vi "GetNameVersion.vi"(8 "error in (no error)":errorcluster, 11 "XML String":string="<?xml version=\"1.0\" encoding=\"utf-8\"?>\n<CustomDevice xmlns:xsi=\"http://www.w3.org/2001/XMLSchema-instance\" xsi:noNamespaceSchemaLocation=\"Custom Device.xsd\">\n<XSDVersion Major=\"2010\" Minor=\"0\" Fix=\"0\" Build=\"0\" />\n  <AddMenu>\n    <eng>NI-XNET Monitor</eng>\n    <loc>NI-XNET Monitor</loc>\n  </AddMenu>\n  <Version>2.0.0</Version>\n  <Type>Inline HW Interface</Type>\n  <MaxOccurrence>1</MaxOccurrence>\n  <MainPageGUID>2fba45b0-1589-4179-a966-5fc49498794e</MainPageGUID>\n  <InitializationVI>\n    <Type>Action</Type>\n    <Item2Launch>\n      <Type>To Common Doc Dir</Type>\n\t\t<Path>Custom Devices\\NI-XNET Monitor\\Windows\\NI-XNET Monitor Configuration.llb\\Initialization VI.vi</Path>\n    </Item2Launch>\n  </InitializationVI>\n  <CustomDeviceVI>\n\t\t<SourceDistribution>\n\t\t\t<Source>\n\t\t\t\t<SupportedTarget>Windows</SupportedTarget>\n\t\t\t\t<Source>\n\t\t\t\t\t<Type>To Common Doc Dir</Type>\n\t\t\t\t\t<Path>Custom Devices\\NI-XNET Monitor\\Windows\\NI-XNET Monitor Engine Windows.llb\\RT Driver VI.vi</Path>\n\t\t\t\t</Source>\n\t\t\t\t<RealTimeSystemDestination>c:\\ni-rt\\VeriStand\\Custom Devices\\NI-XNET Monitor\\NI-XNET Monitor Engine Windows.llb\\RT Driver VI.vi</RealTimeSystemDestination>\n\t\t\t</Source>\n\t\t\t<Source>\n\t\t\t\t<SupportedTarget>Pharlap</SupportedTarget>\n\t\t\t\t<Source>\n\t\t\t\t\t<Type>To Common Doc Dir</Type>\n\t\t\t\t\t<Path>Custom Devices\\NI-XNET Monitor\\PharLap\\NI-XNET Monitor Engine Pharlap.llb\\RT Driver VI.vi</Path>\n\t\t\t\t</Source>\n\t\t\t\t<RealTimeSystemDestination>c:\\ni-rt\\VeriStand\\Custom Devices\\NI-XNET Monitor\\NI-XNET Monitor Engine Pharlap.llb\\RT Driver VI.vi</RealTimeSystemDestination>\n\t\t\t</Source>\n\t\t\t<Source>\n\t\t\t\t<SupportedTarget>VxWorks</SupportedTarget>\n\t\t\t\t<Source>\n\t\t\t\t\t<Type>To Common Doc Dir</Type>\n\t\t\t\t\t<Path>Custom Devices\\NI-XNET Monitor\\VxWorks\\NI-XNET Monitor Engine VxWorks.llb\\RT Driver VI.vi</Path>\n\t\t\t\t</Source>\n\t\t\t\t<RealTimeSystemDestination>c:\\ni-rt\\VeriStand\\Custom Devices\\NI-XNET Monitor\\NI-XNET Monitor Engine VxWorks.llb\\RT Driver VI.vi</RealTimeSystemDestination>\n\t\t\t</Source>\t\n\t\t\t<Source>\n\t\t\t\t<SupportedTarget>Linux_32_ARM</SupportedTarget>\n\t\t\t\t<Source>\n\t\t\t\t\t<Type>To Common Doc Dir</Type>\n\t\t\t\t\t<Path>Custom Devices\\NI-XNET Monitor\\Linux_32_ARM\\NI-XNET Monitor Engine LinuxARM.llb\\RT Driver VI.vi</Path>\n\t\t\t\t</Source>\n\t\t\t\t<RealTimeSystemDestination>c:\\ni-rt\\VeriStand\\Custom Devices\\NI-XNET Monitor\\NI-XNET Monitor Engine LinuxARM.llb\\RT Driver VI.vi</RealTimeSystemDestination>\n\t\t\t</Source>\n\t\t\t<Source>\n\t\t\t\t<SupportedTarget>Linux_x64</SupportedTarget>\n\t\t\t\t<Source>\n\t\t\t\t\t<Type>To Common Doc Dir</Type>\n\t\t\t\t\t<Path>Custom Devices\\NI-XNET Monitor\\Linux_x64\\NI-XNET Monitor Engine Linux64.llb\\RT Driver VI.vi</Path>\n\t\t\t\t</Source>\n\t\t\t\t<RealTimeSystemDestination>c:\\ni-rt\\VeriStand\\Custom Devices\\NI-XNET Monitor\\NI-XNET Monitor Engine Linux64.llb\\RT Driver VI.vi</RealTimeSystemDestination>\n\t\t\t</Source>\n\t\t</SourceDistribution>\n\t</CustomDeviceVI>\n  <Dependencies />\n  <Pages>\n    <Page>\n      <Name>\n        <eng>NI-XNET Monitor</eng>\n        <loc>NI-XNET Monitor</loc>\n      </Name>\n\t  <DisallowRenaming>true</DisallowRenaming>\n      <GUID>2fba45b0-1589-4179-a966-5fc49498794e</GUID>\n      <Glyph>\n\t\t\t<Type>To Common Doc Dir</Type>\n\t\t\t<Path>Custom Devices\\NI-XNET Monitor\\Glyphs\\xnet_monitor.png</Path>\n\t\t</Glyph>\n      <Item2Launch>\n        <Type>To Common Doc Dir</Type>\n\t\t<Path>Custom Devices\\NI-XNET Monitor\\Windows\\NI-XNET Monitor Configuration.llb\\Main Page.vi</Path>\n      </Item2Launch>\n\t  <ButtonList>\n\t\t\t<Button>\n\t\t\t\t<ID>Refresh-Button</ID>\n\t\t\t\t<Glyph>\n\t\t\t\t\t<Type>To Application Data Dir</Type>\n\t\t\t\t\t<Path>System Explorer\\Glyphs\\reload.png</Path>\n\t\t\t\t</Glyph>\n\t\t\t\t<Type>Notification</Type>\n\t\t\t\t<ReferencedGUID>2fba45b0-1589-4179-a966-5fc49498794e</ReferencedGUID>\n\t\t\t\t<ButtonText>\n\t\t\t\t\t<eng>Refresh</eng>\n\t\t\t\t\t<loc>Refresh</loc>\n\t\t\t\t</ButtonText>\n\t\t\t\t<Caption>\n\t\t\t\t\t<eng>Refresh</eng>\n\t\t\t\t\t<loc>Refresh</loc>\n\t\t\t\t</Caption>\n\t\t\t\t<TipStrip>\n\t\t\t\t\t<eng>Refresh NI-XNET channel list</eng>\n\t\t\t\t\t<loc>Refresh NI-XNET channel list</loc>\n\t\t\t\t</TipStrip>\n\t\t\t\t<Documentation>\n\t\t\t\t\t<eng>Refresh NI-XNET channel list</eng>\n\t\t\t\t\t<loc>Refresh NI-XNET channel list</loc>\n\t\t\t\t</Documentation>\n\t\t\t</Button>\n\t  </ButtonList>\n\t  <ActionVIOnDelete>\n \t\t <Type>To Common Doc Dir</Type>\n\t\t <Path>Custom Devices\\NI-XNET Monitor\\Windows\\NI-XNET Monitor Configuration.llb\\ActionVIOnDelete.vi</Path>\n\t  </ActionVIOnDelete>\n      <ActionVIOnLoad>\n        <Type>To Common Doc Dir</Type>\n        <Path>Custom Devices\\NI-XNET Monitor\\Windows\\NI-XNET Monitor Configuration.llb\\ActionVIOnLoad.vi</Path>\n      </ActionVIOnLoad>\n      <ActionVIOnSave>\n        <Type>To Common Doc Dir</Type>\n        <Path>Custom Devices\\NI-XNET Monitor\\Windows\\NI-XNET Monitor Configuration.llb\\ActionVIOnSave.vi</Path>\n      </ActionVIOnSave>\n\t  <ActionVIOnCompile>\n        <Type>To Common Doc Dir</Type>\n        <Path>Custom Devices\\NI-XNET Monitor\\Windows\\NI-XNET Monitor Configuration.llb\\ActionVIOnCompile.vi</Path>\n      </ActionVIOnCompile>\n    </Page>\n    \n<Page>\n      <Name>\n        <eng>Port</eng>\n        <loc>Port</loc>\n      </Name>\n\t  <DisallowRenaming>true</DisallowRenaming>\n\t  <ExcludeFromAlphabeticalOrder>true</ExcludeFromAlphabeticalOrder>\n      <GUID>6e4b4e9f-3d48-4140-aa73-eb1a9ddd4810</GUID>\n      <Glyph>\n\t\t\t<Type>To Application Data Dir</Type>\n\t\t\t<Path>System Explorer\\Glyphs\\NI-XNET Port.png</Path>\n\t\t</Glyph>\n      <Item2Launch>\n        <Type>To Common Doc Dir</Type>\n\t\t<Path>Custom Devices\\NI-XNET Monitor\\Windows\\NI-XNET Monitor Configuration.llb\\Port.vi</Path>\n      </Item2Launch>\n\t  <ButtonList>\n\t\t\t<Button>\n\t\t\t\t<ID>Refresh-Button</ID>\n\t\t\t\t<Glyph>\n\t\t\t\t\t<Type>To Application Data Dir</Type>\n\t\t\t\t\t<Path>System Explorer\\Glyphs\\reload.png</Path>\n\t\t\t\t</Glyph>\n\t\t\t\t<Type>Notification</Type>\n\t\t\t\t<ReferencedGUID>6e4b4e9f-3d48-4140-aa73-eb1a9ddd4810</ReferencedGUID>\n\t\t\t\t<ButtonText>\n\t\t\t\t\t<eng>Refresh</eng>\n\t\t\t\t\t<loc>Refresh</loc>\n\t\t\t\t</ButtonText>\n\t\t\t\t<Caption>\n\t\t\t\t\t<eng>Refresh</eng>\n\t\t\t\t\t<loc>Refresh</loc>\n\t\t\t\t</Caption>\n\t\t\t\t<TipStrip>\n\t\t\t\t\t<eng>Refresh NI-XNET channel list</eng>\n\t\t\t\t\t<loc>Refresh NI-XNET channel list</loc>\n\t\t\t\t</TipStrip>\n\t\t\t\t<Documentation>\n\t\t\t\t\t<eng>Refresh NI-XNET channel list</eng>\n\t\t\t\t\t<loc>Refresh NI-XNET channel list</loc>\n\t\t\t\t</Documentation>\n\t\t\t</Button>\n\t  </ButtonList>\n    </Page>\n<Page>\n      <Name>\n        <eng>Port</eng>\n        <loc>Port</loc>\n      </Name>\n\t  <DisallowRenaming>true</DisallowRenaming>\n\t  <ExcludeFromAlphabeticalOrder>true</ExcludeFromAlphabeticalOrder>\n      <GUID>6e4b4e9f-3d48-4140-aa73-eb1a9ddd4810-DISABLED</GUID>\n      <Glyph>\n\t\t\t<Type>To Application Data Dir</Type>\n\t\t\t<Path>System Explorer\\Glyphs\\NI-XNET Port Disabled.png</Path>\n\t\t</Glyph>\n      <Item2Launch>\n        <Type>To Common Doc Dir</Type>\n\t\t<Path>Custom Devices\\NI-XNET Monitor\\Windows\\NI-XNET Monitor Configuration.llb\\Port.vi</Path>\n      </Item2Launch>\n\t  <ButtonList>\n\t\t\t<Button>\n\t\t\t\t<ID>Refresh-Button</ID>\n\t\t\t\t<Glyph>\n\t\t\t\t\t<Type>To Application Data Dir</Type>\n\t\t\t\t\t<Path>System Explorer\\Glyphs\\reload.png</Path>\n\t\t\t\t</Glyph>\n\t\t\t\t<Type>Notification</Type>\n\t\t\t\t<ReferencedGUID>6e4b4e9f-3d48-4140-aa73-eb1a9ddd4810-DISABLED</ReferencedGUID>\n\t\t\t\t<ButtonText>\n\t\t\t\t\t<eng>Refresh</eng>\n\t\t\t\t\t<loc>Refresh</loc>\n\t\t\t\t</ButtonText>\n\t\t\t\t<Caption>\n\t\t\t\t\t<eng>Refresh</eng>\n\t\t\t\t\t<loc>Refresh</loc>\n\t\t\t\t</Caption>\n\t\t\t\t<TipStrip>\n\t\t\t\t\t<eng>Refresh NI-XNET channel list</eng>\n\t\t\t\t\t<loc>Refresh NI-XNET channel list</loc>\n\t\t\t\t</TipStrip>\n\t\t\t\t<Documentation>\n\t\t\t\t\t<eng>Refresh NI-XNET channel list</eng>\n\t\t\t\t\t<loc>Refresh NI-XNET channel list</loc>\n\t\t\t\t</Documentation>\n\t\t\t</Button>\n\t  </ButtonList>\n    </Page>\n<Page>\n      <Name>\n        <eng>CAN</eng>\n        <loc>CAN</loc>\n      </Name>\n\t  <DisallowRenaming>true</DisallowRenaming>\n\t  <ExcludeFromAlphabeticalOrder>true</ExcludeFromAlphabeticalOrder>\n      <GUID>d0ed4327-8d71-4af7-8daf-159d159a2198</GUID>\n      <Glyph>\n\t\t\t<Type>To Application Data Dir</Type>\n\t\t\t<Path>System Explorer\\Glyphs\\NI-XNET CAN.png</Path>\n\t\t</Glyph>\n      <Item2Launch>\n        <Type>To Common Doc Dir</Type>\n\t\t<Path>Custom Devices\\NI-XNET Monitor\\Windows\\NI-XNET Monitor Configuration.llb\\Interface.vi</Path>\n      </Item2Launch>\n\t  <ButtonList>\n\t\t\t<Button>\n\t\t\t\t<ID>Refresh-Button</ID>\n\t\t\t\t<Glyph>\n\t\t\t\t\t<Type>To Application Data Dir</Type>\n\t\t\t\t\t<Path>System Explorer\\Glyphs\\reload.png</Path>\n\t\t\t\t</Glyph>\n\t\t\t\t<Type>Notification</Type>\n\t\t\t\t<ReferencedGUID>d0ed4327-8d71-4af7-8daf-159d159a2198</ReferencedGUID>\n\t\t\t\t<ButtonText>\n\t\t\t\t\t<eng>Refresh</eng>\n\t\t\t\t\t<loc>Refresh</loc>\n\t\t\t\t</ButtonText>\n\t\t\t\t<Caption>\n\t\t\t\t\t<eng>Refresh</eng>\n\t\t\t\t\t<loc>Refresh</loc>\n\t\t\t\t</Caption>\n\t\t\t\t<TipStrip>\n\t\t\t\t\t<eng>Refresh NI-XNET channel list</eng>\n\t\t\t\t\t<loc>Refresh NI-XNET channel list</loc>\n\t\t\t\t</TipStrip>\n\t\t\t\t<Documentation>\n\t\t\t\t\t<eng>Refresh NI-XNET channel list</eng>\n\t\t\t\t\t<loc>Refresh NI-XNET channel list</loc>\n\t\t\t\t</Documentation>\n\t\t\t</Button>\n\t  </ButtonList>\n    </Page>\n<Page>\n      <Name>\n        <eng>FlexRay</eng>\n        <loc>FlexRay</loc>\n      </Name>\n\t  <DisallowRenaming>true</DisallowRenaming>\n\t  <ExcludeFromAlphabeticalOrder>true</ExcludeFromAlphabeticalOrder>\n      <GUID>b3b15e68-7151-4c2d-a280-06a82878b967</GUID>\n      <Glyph>\n\t\t\t<Type>To Application Data Dir</Type>\n\t\t\t<Path>System Explorer\\Glyphs\\NI-XNET FlexRay.png</Path>\n\t\t</Glyph>\n      <Item2Launch>\n        <Type>To Common Doc Dir</Type>\n\t\t<Path>Custom Devices\\NI-XNET Monitor\\Windows\\NI-XNET Monitor Configuration.llb\\Interface.vi</Path>\n      </Item2Launch>\n\t  <ButtonList>\n\t\t\t<Button>\n\t\t\t\t<ID>Refresh-Button</ID>\n\t\t\t\t<Glyph>\n\t\t\t\t\t<Type>To Application Data Dir</Type>\n\t\t\t\t\t<Path>System Explorer\\Glyphs\\reload.png</Path>\n\t\t\t\t</Glyph>\n\t\t\t\t<Type>Notification</Type>\n\t\t\t\t<ReferencedGUID>b3b15e68-7151-4c2d-a280-06a82878b967</ReferencedGUID>\n\t\t\t\t<ButtonText>\n\t\t\t\t\t<eng>Refresh</eng>\n\t\t\t\t\t<loc>Refresh</loc>\n\t\t\t\t</ButtonText>\n\t\t\t\t<Caption>\n\t\t\t\t\t<eng>Refresh</eng>\n\t\t\t\t\t<loc>Refresh</loc>\n\t\t\t\t</Caption>\n\t\t\t\t<TipStrip>\n\t\t\t\t\t<eng>Refresh NI-XNET channel list</eng>\n\t\t\t\t\t<loc>Refresh NI-XNET channel list</loc>\n\t\t\t\t</TipStrip>\n\t\t\t\t<Documentation>\n\t\t\t\t\t<eng>Refresh NI-XNET channel list</eng>\n\t\t\t\t\t<loc>Refresh NI-XNET channel list</loc>\n\t\t\t\t</Documentation>\n\t\t\t</Button>\n\t  </ButtonList>\n    </Page>\n<Page>\n      <Name>\n        <eng>LIN</eng>\n        <loc>LIN</loc>\n      </Name>\n\t  <DisallowRenaming>true</DisallowRenaming>\n\t  <ExcludeFromAlphabeticalOrder>true</ExcludeFromAlphabeticalOrder>\n      <GUID>c19a2e81-5516-4045-93a5-b1bca7ac20ae</GUID>\n      <Glyph>\n\t\t\t<Type>To Application Data Dir</Type>\n\t\t\t<Path>System Explorer\\Glyphs\\NI-XNET LIN.png</Path>\n\t\t</Glyph>\n      <Item2Launch>\n        <Type>To Common Doc Dir</Type>\n\t\t<Path>Custom Devices\\NI-XNET Monitor\\Windows\\NI-XNET Monitor Configuration.llb\\Interface.vi</Path>\n      </Item2Launch>\n\t  <ButtonList>\n\t\t\t<Button>\n\t\t\t\t<ID>Refresh-Button</ID>\n\t\t\t\t<Glyph>\n\t\t\t\t\t<Type>To Application Data Dir</Type>\n\t\t\t\t\t<Path>System Explorer\\Glyphs\\reload.png</Path>\n\t\t\t\t</Glyph>\n\t\t\t\t<Type>Notification</Type>\n\t\t\t\t<ReferencedGUID>c19a2e81-5516-4045-93a5-b1bca7ac20ae</ReferencedGUID>\n\t\t\t\t<ButtonText>\n\t\t\t\t\t<eng>Refresh</eng>\n\t\t\t\t\t<loc>Refresh</loc>\n\t\t\t\t</ButtonText>\n\t\t\t\t<Caption>\n\t\t\t\t\t<eng>Refresh</eng>\n\t\t\t\t\t<loc>Refresh</loc>\n\t\t\t\t</Caption>\n\t\t\t\t<TipStrip>\n\t\t\t\t\t<eng>Refresh NI-XNET channel list</eng>\n\t\t\t\t\t<loc>Refresh NI-XNET channel list</loc>\n\t\t\t\t</TipStrip>\n\t\t\t\t<Documentation>\n\t\t\t\t\t<eng>Refresh NI-XNET channel list</eng>\n\t\t\t\t\t<loc>Refresh NI-XNET channel list</loc>\n\t\t\t\t</Documentation>\n\t\t\t</Button>\n\t  </ButtonList>\n    </Page>\n<Page>\n      <Name>\n        <eng>PortStatus</eng>\n        <loc>PortStatus</loc>\n      </Name>\n\t  <DisallowRenaming>true</DisallowRenaming>\n\t  <ExcludeFromAlphabeticalOrder>true</ExcludeFromAlphabeticalOrder>\n      <GUID>20dbf2c1-039f-4944-a9cd-53b00268baa8</GUID>\n      <Glyph>\n\t\t\t<Type>To Application Data Dir</Type>\n\t\t\t<Path>System Explorer\\Glyphs\\system variable.png</Path>\n\t\t</Glyph>\n      <Item2Launch>\n        <Type>To Common Doc Dir</Type>\n\t\t<Path>Custom Devices\\NI-XNET Monitor\\Windows\\NI-XNET Monitor Configuration.llb\\PortChannel.vi</Path>\n      </Item2Launch>\n    </Page>\n<Page>\n      <Name>\n        <eng>PortError</eng>\n        <loc>PortError</loc>\n      </Name>\n\t  <DisallowRenaming>true</DisallowRenaming>\n\t  <ExcludeFromAlphabeticalOrder>true</ExcludeFromAlphabeticalOrder>\n      <GUID>37c19a15-61f7-4078-98c8-bfb7f6b25de3</GUID>\n      <Glyph>\n\t\t\t<Type>To Application Data Dir</Type>\n\t\t\t<Path>System Explorer\\Glyphs\\NI-XNET TransceiverState.png</Path>\n\t\t</Glyph>\n      <Item2Launch>\n        <Type>To Common Doc Dir</Type>\n\t\t<Path>Custom Devices\\NI-XNET Monitor\\Windows\\NI-XNET Monitor Configuration.llb\\PortChannel.vi</Path>\n      </Item2Launch>\n    </Page>\n  </Pages>\n  <CustomXML>\n    <Dummy></Dummy>\n  </CustomXML>\n</CustomDevice>") -> (0 "error out":errorcluster, 2 "Custom Device Version":string, 3 "Custom Device Name":string)   [LabVIEW 2020, in "Shared.lvlib"]
uses:
  Shared.lvlib
  <vilib>/xml/Load XML String.vi
  <vilib>/xml/Close Reference(Node).vi
  <vilib>/xml/NI_XML.lvlib
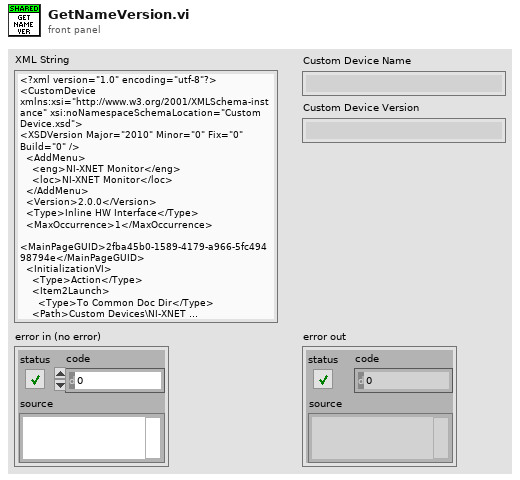
[diagram p1: front panel]
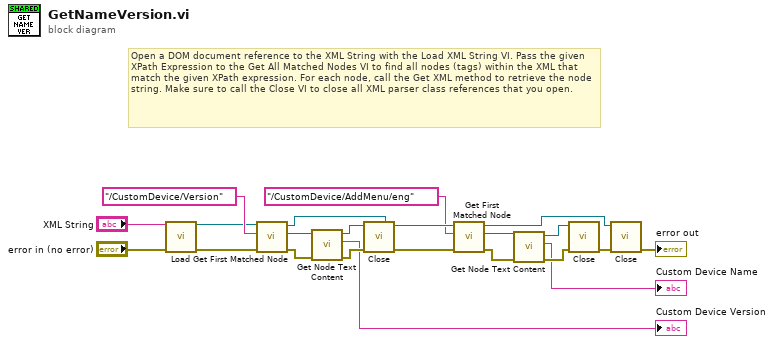
[diagram p0: block diagram]
diagram:
  # "Open a DOM document reference to the XML String with the Load XML String VI. Pass the given XPath Expression to the Get All Matched Nodes VI to find all nodes (tags) within the XML that match the given XPath expression. For each node, call the Get XML method to retrieve the node string. Make sure to call the Close VI to close all XML parser class references that you open."
  n1 = call-poly <vilib>:"Load.vi"("XML string"="XML String", "error in (no error)"="error in (no error)") -> ("DOM document out"=w20:refnum<k20>, "error out"=w19:errorcluster)  [unwired: 11 in, 1 out]
  n2 = call <vilib>:"Get First Matched Node.vi"("error in (no error)"=w19, "XPath expression"="/CustomDevice/Version" ("XPath Expression"), "node in"=w20) -> ("error out"=w8:errorcluster, "node result"=w10:refnum<k20>, "node out"=w15:refnum<k20>)  [unwired: 6 in]
  n3 = call <vilib>:"Get Node Text Content.vi"("error in (no error)"=w8, "node in"=w10) -> ("error out"=w9:errorcluster, "node text"=→"Custom Device Version":string, "node out"=w6:refnum<k20>)  [unwired: 7 in]
  n4 = call-poly <vilib>:"Close.vi"("error in (no error)"=w9, "node"=w6) -> ("error out"=w14:errorcluster)  [unwired: 7 out]
  n5 = call <vilib>:"Get First Matched Node.vi"("error in (no error)"=w14, "XPath expression"="/CustomDevice/AddMenu/eng" ("XPath Expression"), "node in"=w15) -> ("error out"=w4:errorcluster, "node result"=w5:refnum<k20>, "node out"=w11:refnum<k20>)  [unwired: 6 in]
  n6 = call <vilib>:"Get Node Text Content.vi"("error in (no error)"=w4, "node in"=w5) -> ("error out"=w2:errorcluster, "node text"=→"Custom Device Name":string, "node out"=w3:refnum<k20>)  [unwired: 7 in]
  n7 = call-poly <vilib>:"Close.vi"("error in (no error)"=w2, "node"=w3) -> ("error out"=w12:errorcluster)  [unwired: 7 out]
  n8 = call-poly <vilib>:"Close.vi"("error in (no error)"=w12, "node"=w11) -> ("error out"=→"error out":errorcluster)  [unwired: 7 out]
